vi "Check_duration.vi"(10 "Duration":i32, 11 "CT1":timestamp) -> (3 "Initial State":T1)   [LabVIEW 2015]
uses:
  C:/Program Files (x86)/National Instruments/LabVIEW 2015/examples/Data Communication/Protocols/TCP/TCP Multiple Connections/controls/TCP Multiple Connections State.ctl
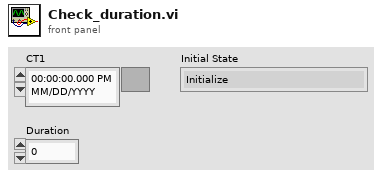
[diagram p1: front panel]
types:
  T1 = typedef "TCP Multiple Connections State.ctl" = enum16{"Initialize", "Status Check", "Measurement", "Return Values to DEV", "Stop"}
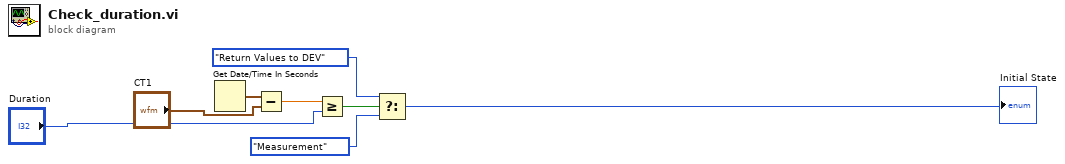
[diagram p0: block diagram]
diagram:
  n1 = Get Date/Time In Seconds() -> (seconds since 1Jan1904=w1:timestamp)
  n2 = Subtract(x=w1, y="CT1") -> (x-y=w3:dbl)
  n3 = Greater Or Equal?(x=w3, y="Duration") -> (x >= y?=w5:bool)
  n4 = Select(t=TCP_Multiple_Connections_State."Return Values to DEV" ("Initial State"), s=w5, f=TCP_Multiple_Connections_State."Measurement" ("Initial State")) -> (s? t:f=→"Initial State":T1)
